vi "Begin.vi"(8 "error in":errorcluster) -> (0 "error out":errorcluster)   [LabVIEW 2015]
doc: "Called before other user functions, this VI is expected to open initial I/O refnums, load in file data, and do all program initialization. Notice that the <B>error out</B> terminal is simply used for data flow. Wiring it to other structures or subVIs ensures that this VI runs first."
uses:
  <vilib>/Rock Robotics/WPI/DriverStation/WPI_DriverStationRobotMode2.ctl
  <vilib>/Rock Robotics/WPI/Joystick/WPI_JoystickDeviceEnum.ctl
  <vilib>/Rock Robotics/SystemInterfaces/DIO/FPGA_DIOPWMChannel.ctl
  <vilib>/Rock Robotics/WPI/Camera/WPI_CameraWhite Balance Values.ctl
  <vilib>/Rock Robotics/WPI/Camera/WPI_CameraExposure Values.ctl
  <vilib>/Rock Robotics/WPI/Camera/WPI_CameraFrameRate.ctl
  <vilib>/Rock Robotics/WPI/Camera/WPI_CameraImageSize.ctl
  Robot Global Data.vi
  <vilib>/Rock Robotics/Network Tables/NT Write String Array.vi
  <vilib>/Rock Robotics/WPI/MotorControl/WPI_MotorControlOpen Talon.vi
  <vilib>/Rock Robotics/WPI/MotorControl/WPI_MotorControlOpen Victor.vi
  SubSystems/References/Refnums.vi
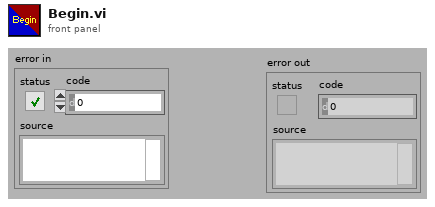
[diagram p1: front panel]
types:
  T1 = typedef "WPI_CameraImageSize.ctl" = enum16{"640x480", "320x240", "160x120", "Custom"}
  T2 = typedef "WPI_CameraFrameRate.ctl" = u32
  T3 = typedef "WPI_CameraExposure Values.ctl" = enum16{"Auto", "Flicker-free 50 Hz", "Flicker-free 60 Hz", "Hold current", "Custom"}
  T4 = typedef "WPI_CameraWhite Balance Values.ctl" = enum16{"Auto", "Fixed indoor", "Fixed outdoor 1", "Fixed outdoor 2", "Fixed fluorescent 1", "Fixed fluorescent 2", "Hold current", "Custom"}
  T5 = typedef "FPGA_DIOPWMChannel.ctl" = enum8{"PWM 0", "PWM 1", "PWM 2", "PWM 3", "PWM 4", "PWM 5", "PWM 6", "PWM 7", "PWM 8", "PWM 9", "PWM MXP 0", "PWM MXP 1", "PWM MXP 2", "PWM MXP 3", "PWM MXP 4", "PWM MXP 5", "PWM MXP 6", "PWM MXP 7", "PWM MXP 8", "PWM MXP 9", "Invalid"}
  T6 = typedef "WPI_JoystickDeviceEnum.ctl" = enum16{"USB 0", "USB 1", "USB 2", "USB 3", "USB 4", "USB 5"}
  T7 = typedef "WPI_DriverStationRobotMode2.ctl" = enum16{"Autonomous Disabled", "Autonomous Enabled", "Teleop Disabled", "Teleop Enabled", "Disconnected", "Finish", "Test Disabled", "Test Enabled", "Emergency Stopped"}
  T8 = typedef "WPI_JoystickDevRef.ctl" = cluster{"Device":T6}
  T9 = typedef "WPI_CameraDevRef.ctl" = cluster{"Camera Address":string, "CameraStatus":errorcluster}
  T10 = typedef "WPI_MotorControlDeviceRef.ctl" = cluster{"DeviceStatus":errorcluster, "Type":T11, "PWM":cluster{"PWM Channel":T5, "DeadBand":T12}, "CAN":cluster{"Device Number":u8, "Control Mode":T13, "Semaphore":T14, "Max Vout":dbl, "TalonSRX Control Mode":T15}, "Invert":bool}
  T11 = typedef "WPI_MotorControlType.ctl" = enum16{"PWM", "CAN", "CANTalonSRX"}
  T12 = typedef "WPI_PWMDeadband.ctl" = cluster{"Name":string, "maxPositivePwm":i32, "minPositivePwm":i32, "centerPwm":i32, "maxNegativePwm":i32, "minNegativePwm":i32, "angularRange":u16}
  T13 = typedef "WPI_CANJaguar_ControlMode.ctl" = enum8{"Percent VBus", "Current", "Speed", "Position", "Voltage"}
  T14 = typedef "Semaphore RefNum" = refnum<k1>
  T15 = typedef "WPI_CANTalonSRX_APIControlMode.ctl" = enum8{"Percent VBus", "Speed", "Position", "Slave", "Unchanged / Invalid", "Voltage Compensation", "Current", "Motion Profile"}
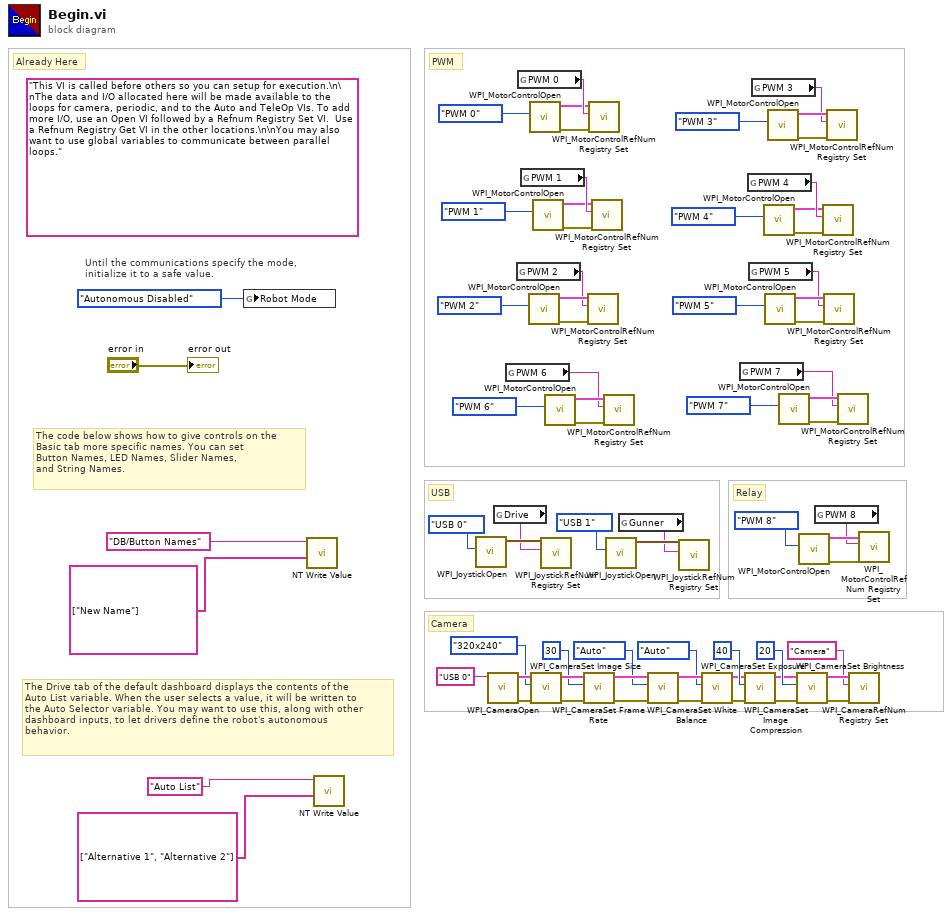
[diagram p0: block diagram]
diagram:
  (unwired) "This VI is called before others so you can setup for execution.\n\nThe data and I/O allocated here will be made available to the loops for camera, periodic, and to the Auto and TeleOp VIs. To add more I/O, use an Open VI followed by a Refnum Registry Set VI.  Use a Refnum Registry Get VI in the other locations.\n\nYou may also want to use global variables to communicate between parallel loops."
  # "Camera"
  # "PWM"
  # "Already Here"
  # "USB"
  # "Relay"
  # "The Drive tab of the default dashboard displays the contents of the\nAuto List variable. When the user selects a value, it will be written to\nthe Auto Selector variable. You may want to use this, along with other\ndashboard inputs, to let drivers define the robot's autonomous\nbehavior."
  # "The code below shows how to give controls on the\nBasic tab more specific names. You can set\nButton Names, LED Names, Slider Names,\nand String Names."
  # "Until the communications specify the mode,\ninitialize it to a safe value."
  n1 = global write "Robot Global Data.vi" "Robot Mode"(WPI_DriverStationRobotMode2."Autonomous Disabled" ("Robot Mode")) -> ()
  n2 = call-poly <vilib>:"NT Write Value.vi"("String Array"=string[] ["New Name"], "Name"="DB/Button Names") -> ()  [unwired: 9 in, 1 out]
  n3 = call-poly <vilib>:"NT Write Value.vi"("String Array"=string[] ["Alternative 1", "Alternative 2"], "Name"="Auto List") -> ()  [unwired: 9 in, 1 out]
  n4 = call <vilib>:"WPI_JoystickOpen.vi"("JoystickDevice"=WPI_JoystickDeviceEnum."USB 0") -> ("JoystickDevRef"=w64:T8)  [unwired: 10 in]
  n5 = call <vilib>:"WPI_CameraOpen.vi"("Camera Address"="USB 0" ("format string")) -> ("error out"=w12:errorcluster, "CameraDevRef"=w13:T9)  [unwired: 1 in, 8 out]
  n6 = global read "Refnums.vi" "Drive"() -> (w62:string)
  n7 = global read "Refnums.vi" "PWM 6"() -> (w51:string)
  n8 = global read "Refnums.vi" "PWM 2"() -> (w30:string)
  n9 = global read "Refnums.vi" "PWM 0"() -> (w38:string)
  n10 = global read "Refnums.vi" "PWM 1"() -> (w34:string)
  n11 = call-poly <vilib>:"WPI_MotorControlOpen.vi"("PWM Channel"=FPGA_DIOPWMChannel."PWM 2") -> ("error out"=w29:errorcluster, "MotorControlDeviceRef"=w31:T10)  [unwired: 9 in]
  n12 = call-poly <vilib>:"WPI_MotorControlOpen.vi"("PWM Channel"=FPGA_DIOPWMChannel."PWM 0") -> ("error out"=w35:errorcluster, "MotorControlDeviceRef"=w37:T10)  [unwired: 9 in]
  n13 = call <vilib>:"WPI_CameraSet Image Size.vi"("error in (no error)"=w12, "Image Size"=WPI_CameraImageSize."320x240", "CameraDevRef"=w13) -> ("error out"=w11:errorcluster, "CameraDevRef Out"=w14:T9)  [unwired: 1 in, 6 out]
  n14 = call-poly <vilib>:"WPI_MotorControlOpen.vi"("PWM Channel"=FPGA_DIOPWMChannel."PWM 1") -> ("error out"=w32:errorcluster, "MotorControlDeviceRef"=w33:T10)  [unwired: 9 in]
  n15 = call <vilib>:"WPI_JoystickRefNum Registry Set.vi"("refnum name"=w62, "JoystickDevRef"=w64) -> ()  [unwired: 8 in, 2 out]
  n16 = call-poly <vilib>:"WPI_MotorControlOpen.vi"("PWM Channel"=FPGA_DIOPWMChannel."PWM 6") -> ("error out"=w53:errorcluster, "MotorControlDeviceRef"=w52:T10)  [unwired: 9 in]
  n17 = call <vilib>:"WPI_CameraSet Frame Rate.vi"("error in (no error)"=w11, "Frame Rate (fps)"=T2 30, "CameraDevRef"=w14) -> ("error out"=w10:errorcluster, "CameraDevRef Out"=w16:T9)  [unwired: 7 out]
  n18 = call <vilib>:"WPI_MotorControlRefNum Registry Set.vi"("error in (no error)"=w29, "refnum name"=w30, "MotorControlDevRef"=w31) -> ()  [unwired: 7 in, 2 out]
  n19 = call <vilib>:"WPI_MotorControlRefNum Registry Set.vi"("error in (no error)"=w35, "refnum name"=w38, "MotorControlDevRef"=w37) -> ()  [unwired: 7 in, 2 out]
  n20 = call <vilib>:"WPI_MotorControlRefNum Registry Set.vi"("error in (no error)"=w32, "refnum name"=w34, "MotorControlDevRef"=w33) -> ()  [unwired: 7 in, 2 out]
  n21 = call <vilib>:"WPI_MotorControlRefNum Registry Set.vi"("error in (no error)"=w53, "refnum name"=w51, "MotorControlDevRef"=w52) -> ()  [unwired: 7 in, 2 out]
  n22 = call <vilib>:"WPI_JoystickOpen.vi"("JoystickDevice"=WPI_JoystickDeviceEnum."USB 1") -> ("JoystickDevRef"=w63:T8)  [unwired: 10 in]
  n23 = global read "Refnums.vi" "Gunner"() -> (w61:string)
  n24 = call <vilib>:"WPI_CameraSet White Balance.vi"("error in (no error)"=w10, "White Balance"=WPI_CameraWhite_Balance_Values."Auto", "CameraDevRef"=w16) -> ("error out"=w9:errorcluster, "CameraDevRef Out"=w15:T9)  [unwired: 1 in, 6 out]
  n25 = call <vilib>:"WPI_JoystickRefNum Registry Set.vi"("refnum name"=w61, "JoystickDevRef"=w63) -> ()  [unwired: 8 in, 2 out]
  n26 = call <vilib>:"WPI_CameraSet Exposure.vi"("error in (no error)"=w9, "Exposure"=WPI_CameraExposure_Values."Auto", "CameraDevRef"=w15) -> ("error out"=w8:errorcluster, "CameraDevRef Out"=w18:T9)  [unwired: 1 in, 6 out]
  n27 = global read "Refnums.vi" "PWM 7"() -> (w54:string)
  n28 = call <vilib>:"WPI_CameraSet Image Compression.vi"("error in (no error)"=w8, "Compression"=40, "CameraDevRef"=w18) -> ("error out"=w7:errorcluster, "CameraDevRef Out"=w17:T9)  [unwired: 7 out]
  n29 = global read "Refnums.vi" "PWM 4"() -> (w43:string)
  n30 = global read "Refnums.vi" "PWM 5"() -> (w39:string)
  n31 = global read "Refnums.vi" "PWM 3"() -> (w44:string)
  n32 = call-poly <vilib>:"WPI_MotorControlOpen.vi"("PWM Channel"=FPGA_DIOPWMChannel."PWM 4") -> ("error out"=w41:errorcluster, "MotorControlDeviceRef"=w42:T10)  [unwired: 9 in]
  n33 = call-poly <vilib>:"WPI_MotorControlOpen.vi"("PWM Channel"=FPGA_DIOPWMChannel."PWM 5") -> ("error out"=w36:errorcluster, "MotorControlDeviceRef"=w40:T10)  [unwired: 9 in]
  n34 = call-poly <vilib>:"WPI_MotorControlOpen.vi"("PWM Channel"=FPGA_DIOPWMChannel."PWM 3") -> ("error out"=w45:errorcluster, "MotorControlDeviceRef"=w46:T10)  [unwired: 9 in]
  n35 = call-poly <vilib>:"WPI_MotorControlOpen.vi"("PWM Channel"=FPGA_DIOPWMChannel."PWM 7") -> ("error out"=w56:errorcluster, "MotorControlDeviceRef"=w55:T10)  [unwired: 9 in]
  n36 = call <vilib>:"WPI_CameraSet Brightness.vi"("error in (no error)"=w7, "Brightness"=20, "CameraDevRef"=w17) -> ("error out"=w6:errorcluster, "CameraDevRef Out"=w22:T9)  [unwired: 7 out]
  n37 = call-poly <vilib>:"WPI_MotorControlOpen.vi"("PWM Channel"=FPGA_DIOPWMChannel."PWM 8") -> ("error out"=w49:errorcluster, "MotorControlDeviceRef"=w48:T10)  [unwired: 9 in]
  n38 = global read "Refnums.vi" "PWM 8"() -> (w47:string)
  n39 = call <vilib>:"WPI_MotorControlRefNum Registry Set.vi"("error in (no error)"=w41, "refnum name"=w43, "MotorControlDevRef"=w42) -> ()  [unwired: 7 in, 2 out]
  n40 = call <vilib>:"WPI_MotorControlRefNum Registry Set.vi"("error in (no error)"=w36, "refnum name"=w39, "MotorControlDevRef"=w40) -> ()  [unwired: 7 in, 2 out]
  n41 = call <vilib>:"WPI_MotorControlRefNum Registry Set.vi"("error in (no error)"=w45, "refnum name"=w44, "MotorControlDevRef"=w46) -> ()  [unwired: 7 in, 2 out]
  n42 = call <vilib>:"WPI_MotorControlRefNum Registry Set.vi"("error in (no error)"=w56, "refnum name"=w54, "MotorControlDevRef"=w55) -> ()  [unwired: 7 in, 2 out]
  n43 = call <vilib>:"WPI_CameraRefNum Registry Set.vi"("error in (no error)"=w6, "refnum name"="Camera", "CameraDevRef"=w22) -> ()  [unwired: 1 in, 8 out]
  n44 = call <vilib>:"WPI_MotorControlRefNum Registry Set.vi"("error in (no error)"=w49, "refnum name"=w47, "MotorControlDevRef"=w48) -> ()  [unwired: 7 in, 2 out]
  "error out" <- "error in"
